vi "sequence_convertor.vi"(10 "Sequence":string) -> (0 "Sequence(Chr)":string[](array[string]), 2 "Sequence(Num)":i32[](array[numeric]), 3 "Length":i32)   [LabVIEW 2012]
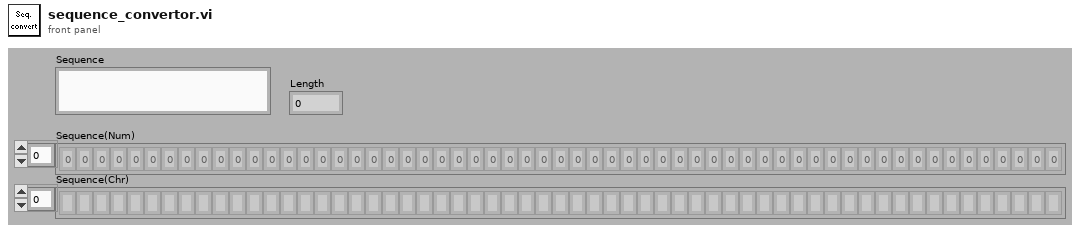
[diagram p1: front panel]
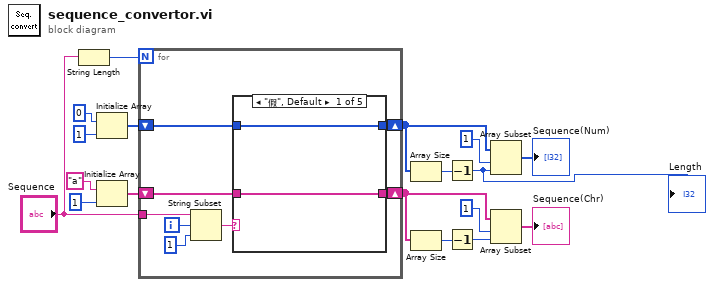
[diagram p0: block diagram]
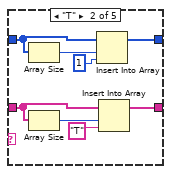
[diagram p2: hidden frame]
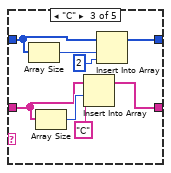
[diagram p3: hidden frame]
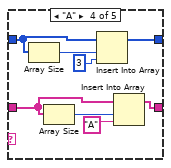
[diagram p4: hidden frame]
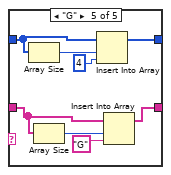
[diagram p5: hidden frame]
diagram:
  n1 = String Length(string="Sequence") -> (length=w17:i32)
  n2 = Initialize Array(u8 0 ("元素"), 1 ("维数大小")) -> (w14:u8[])
  n3 = Initialize Array("a", 1 ("维数大小")) -> (w8:string[])
  n4 = for {
    N: w17 -> [_]
    tunnel: "Sequence" -> [w26]
    shift-right: [w21] -> w12
    shift-left: w14 -> [w22]
    shift-right: [w19] -> w2
    shift-left: w8 -> [w20]
    i -> [w25]
    n5 = String Subset(string=w26, offset (0)=w25, length (rest)=1 ("长度（剩余）")) -> (substring=w23:string)
    n6 = case shown="\"假\", Default" w23 {
      tunnel: w22 -> [w28 w34 w43 w50 w59]
      tunnel: [w28 w35 w42 w51 w60] -> w21
      tunnel: w20 -> [w27 w31 w38 w46 w53]
      tunnel: [w27 w30 w37 w45 w54] -> w19
      frame "假", Default {
      }
      frame "T" {
        n7 = Array Size(array=w34) -> (size(s)=w33:i32)
        n8 = Array Size(array=w31) -> (size(s)=w32:i32)
        n9 = Insert Into Array(array=w34, index=w33, new element=1) -> (w35:u8[])
        n10 = Insert Into Array(array=w31, index=w32, new element="T") -> (w30:string[])
      }
      frame "C" {
        n11 = Array Size(array=w43) -> (size(s)=w41:i32)
        n12 = Array Size(array=w38) -> (size(s)=w40:i32)
        n13 = Insert Into Array(array=w38, index=w40, new element="C") -> (w37:string[])
        n14 = Insert Into Array(array=w43, index=w41, new element=2) -> (w42:u8[])
      }
      frame "A" {
        n15 = Array Size(array=w50) -> (size(s)=w49:i32)
        n16 = Array Size(array=w46) -> (size(s)=w48:i32)
        n17 = Insert Into Array(array=w50, index=w49, new element=3) -> (w51:u8[])
        n18 = Insert Into Array(array=w46, index=w48, new element="A") -> (w45:string[])
      }
      frame "G" {
        n19 = Array Size(array=w59) -> (size(s)=w57:i32)
        n20 = Array Size(array=w53) -> (size(s)=w56:i32)
        n21 = Insert Into Array(array=w59, index=w57, new element=4) -> (w60:u8[])
        n22 = Insert Into Array(array=w53, index=w56, new element="G") -> (w54:string[])
      }
    }
  }
  n23 = Array Size(array=w12) -> (size(s)=w11:i32)
  n24 = Array Size(array=w2) -> (size(s)=w4:i32)
  n25 = Decrement(x=w11) -> (x-1=w1:i32)
  "Length" <- w1
  n26 = Decrement(x=w4) -> (x-1=w5:i32)
  n27 = Array Subset(array=w12, index=1 ("索引"), length=w1) -> (→"Sequence(Num)":u8[])
  n28 = Array Subset(array=w2, index=1 ("索引"), length=w5) -> (→"Sequence(Chr)":string[])
